vi "Create.vi"(8 "error in (no error)":errorcluster, 10 "MsgQ":refnum<class "MessageQ.lvclass">) -> (0 "error out":errorcluster, 3 "HTTPCmdController out":refnum<class "HTTPCmdController.lvclass">)   [LabVIEW 2020, in "Volatus.lvlib" / "HTTPCmdController.lvclass"]
uses:
  HTTPCmdController.lvclass
  HTTPCmdController.lvclass/HTTPCmdController.ctl
  MessageQ/MessageQ.lvclass
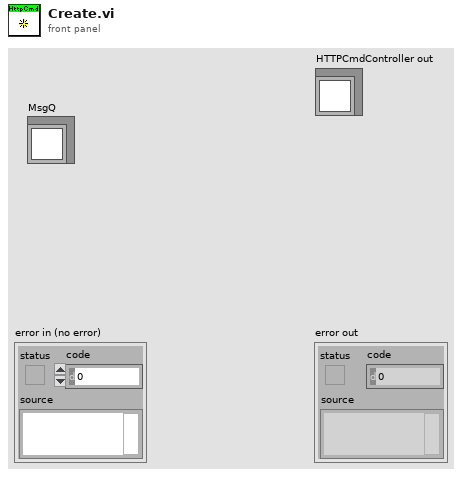
[diagram p1: front panel]
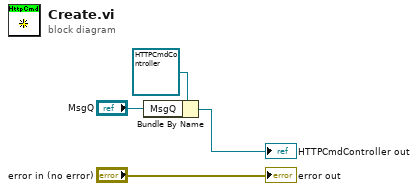
[diagram p0: block diagram]
diagram:
  n1 = Bundle By Name(cluster=refnum<class "HTTPCmdController.lvclass"> refnum ("HTTPCmdController in"), "MsgQ"="MsgQ") -> (→"HTTPCmdController out":refnum<class "HTTPCmdController.lvclass">)
  "error out" <- "error in (no error)"
